vi "FringeTracker-Scan.vi"(7 "FringeTrackerData":T3={"Readout"={"Readout"=100, "Deglitch"=10, "Framerate"=200.0, "Bank"=2}, "Wavelength"=2.2e-06, "Frame per fringe"=5.0, "Autcollimation"=TRUE, "OPD stroke"=0.0, "OPD per pixel"=0.0, "Offset"=0.0} {"Offset" format="%.6g"; "Frame per fringe" format="%.2f"; "Wavelength" format="%.2f"}, 8 "error in (no error)":errorcluster) -> (0 "error out":errorcluster, 5 "FringeTrackerInfo":T1={"Readout"={"Readout"=100, "Deglitch"=10, "Framerate"=200.0, "Bank"=2}, "OPD stroke"=0.0, "OPD per pixel"=0.0})   [LabVIEW 2009]
uses:
  Controls/FringeTrackerData.ctl
  Nicmos/Controls/NICMOS.READOUT.ctl
  Controls/FringeTrackerInfo.ctl
  Controls/FringTrackerCommand.ctl
  Controls/FringeTrackerState.ctl
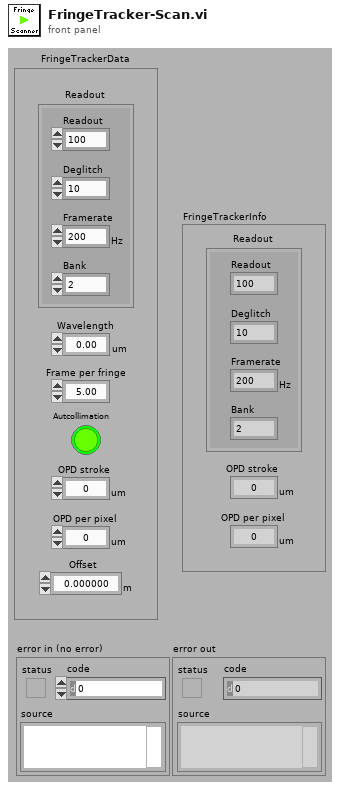
[diagram p1: front panel]
types:
  T1 = typedef "FringeTrackerInfo.ctl" = cluster{"Readout":T2, "OPD stroke":dbl[unit], "OPD per pixel":dbl[unit]}
  T2 = typedef "NICMOS.READOUT.ctl" = cluster{"Readout":i32, "Deglitch":i32, "Framerate":dbl[unit], "Bank":i32}
  T3 = typedef "FringeTrackerData.ctl" = cluster{"Readout":T2, "Wavelength":dbl[unit], "Frame per fringe":dbl, "Autcollimation":bool, "OPD stroke":dbl[unit], "OPD per pixel":dbl[unit], "Offset":dbl[unit]}
  T4 = typedef "FringeTrackerState.ctl" = enum16{"IDLING", "CONFIGURING", "SCANNING", "SEARCHING", "TRACKING", "STOPPING"}
  T5 = typedef "FringTrackerCommand.ctl" = cluster{"Command":enum16{"IDLE", "SCAN", "TRACK", "QUIT"}, "FringeTrackerData":T3}
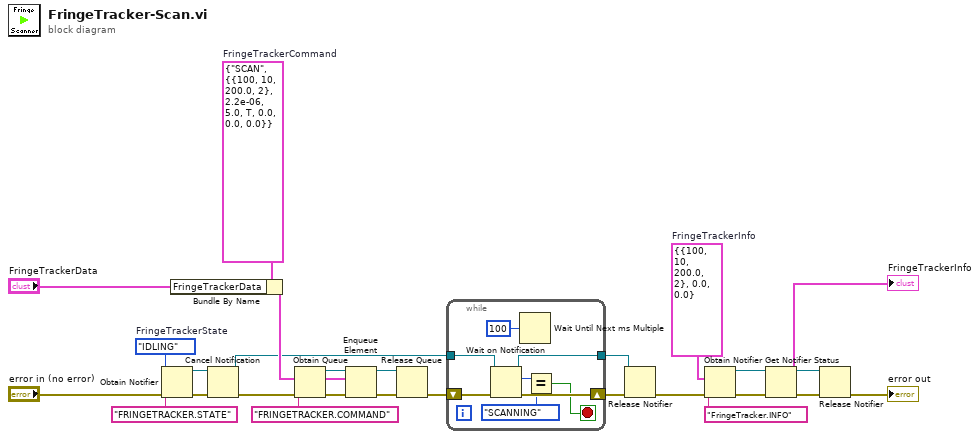
[diagram p0: block diagram]
diagram:
  w14 = FringeTrackerState."IDLING"  # FringeTrackerState
  w21 = T1 {"Readout"={"Readout"=100, "Deglitch"=10, "Framerate"=200.0, "Bank"=2}, "OPD stroke"=0.0, "OPD per pixel"=0.0}  # FringeTrackerInfo
  w26 = T5 {"Command"=enum."SCAN", "FringeTrackerData"={"Readout"={"Readout"=100, "Deglitch"=10, "Framerate"=200.0, "Bank"=2}, "Wavelength"=2.2e-06, "Frame per fringe"=5.0, "Autcollimation"=TRUE, "OPD stroke"=0.0, "OPD per pixel"=0.0, "Offset"=0.0}}  # FringeTrackerCommand
  n1 = Obtain Notifier(name (unnamed)="FRINGETRACKER.STATE", notification data type=w14, error in (no error)="error in (no error)") -> (notifier out=w8:refnum<notifier>, error out=w10:errorcluster)  [unwired: 1 in, 1 out]
  n2 = Bundle By Name(cluster=w26, "FringeTrackerData"="FringeTrackerData") -> (w11:T5)
  n3 = Cancel Notification(0:w8, 3:w10) -> (8:w7:refnum<notifier>, 11:w9:errorcluster)  [unwired: 1 out]
  n4 = Obtain Queue(name (unnamed)="FRINGETRACKER.COMMAND", element data type=w11, error in (no error)=w9) -> (queue out=w23:refnum<queue>, error out=w24:errorcluster)  [unwired: 2 in, 1 out]
  n5 = Enqueue Element(queue=w23, element=w11, error in (no error)=w24) -> (queue out=w6:refnum<queue>, error out=w5:errorcluster)  [unwired: 1 in, 1 out]
  n6 = Release Queue(queue=w6, error in (no error)=w5) -> (error out=w4:errorcluster)  [unwired: 1 in, 2 out]
  n7 = while {
    shift-right: [w34] -> w3
    shift-left: w4 -> [w35]
    tunnel: w7 -> [w29]
    tunnel: [w28] -> w2
    stop <- w31 stop-if-true
    n8 = Wait on Notification(notifier=w29, error in (no error)=w35) -> (notifier out=w28:refnum<notifier>, notification=w33:T4, error out=w34:errorcluster)  [unwired: 2 in, 1 out]
    n9 = Wait Until Next ms Multiple(millisecond multiple=u32 100) -> ()  [unwired: 1 out]
    n10 = Equal?(x=w33, y=FringeTrackerState."SCANNING" ("notification")) -> (x = y?=w31:bool)
  }
  n11 = Release Notifier(notifier=w2, error in (no error)=w3) -> (error out=w1:errorcluster)  [unwired: 1 in, 2 out]
  n12 = Obtain Notifier(name (unnamed)="FringeTracker.INFO", notification data type=w21, error in (no error)=w1) -> (notifier out=w17:refnum<notifier>, error out=w16:errorcluster)  [unwired: 1 in, 1 out]
  n13 = Get Notifier Status(notifier=w17, error in (no error)=w16) -> (notifier out=w19:refnum<notifier>, current notification=→"FringeTrackerInfo":T1, error out=w20:errorcluster)  [unwired: 2 out]
  n14 = Release Notifier(notifier=w19, error in (no error)=w20) -> (error out=→"error out":errorcluster)  [unwired: 1 in, 2 out]
